vi "Read Digital IO Port.vi"(8 "error in (no error)":errorcluster, 11 "VISA resource name":refnum<visa-resource-name>) -> (0 "error out":errorcluster, 2 "Digital IO Value":i32, 3 "VISA resource name out":refnum<visa-resource-name>)   [LabVIEW 2016, in "Keithley DMM7510.lvlib"]
doc: "Reads the digital I/O port."
uses:
  Keithley DMM7510.lvlib
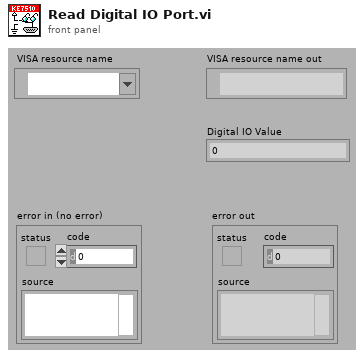
[diagram p1: front panel]
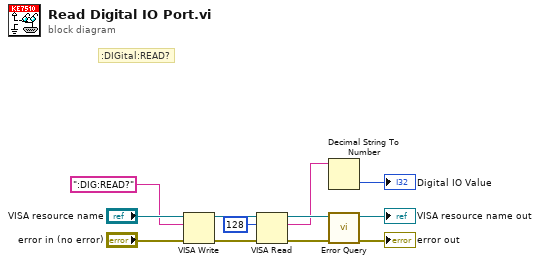
[diagram p0: block diagram]
diagram:
  # ":DIGital:READ?"
  n1 = VISA Write(VISA resource name="VISA resource name", write buffer=":DIG:READ?" ("format string"), error in (no error)="error in (no error)") -> (VISA resource name out=w6:refnum<visa-resource-name>, error out=w4:errorcluster)  [unwired: 1 out]
  n2 = VISA Read(VISA resource name=w6, byte count=u32 128, error in (no error)=w4) -> (VISA resource name out=w5:refnum<visa-resource-name>, read buffer=w2:string, error out=w3:errorcluster)  [unwired: 1 out]
  n3 = Decimal String To Number(string=w2) -> (number=→"Digital IO Value":i32)  [unwired: 2 in, 1 out]
  n4 = call "Error Query.vi"("error in (no error)"=w3, "VISA resource name"=w5) -> ("error out"=→"error out":errorcluster, "VISA resource name out"=→"VISA resource name out":refnum<visa-resource-name>)  [unwired: 6 in, 2 out]
